vi "Actor Core.vi"(8 "error in":errorcluster, 11 "On-Grid in":refnum<class "On-Grid.lvclass">) -> (0 "error out":errorcluster, 3 "Actor out":refnum<class "Actor.lvclass">)   [LabVIEW 2018, in "On-Grid Actor.lvlib" / "On-Grid.lvclass"]
doc: "(<B>Filename</B>: Actor Framework.lvlib:Actor.lvclass:Actor Core.vi)\n\nReceives messages to the actor, reacts to them, and initiates any error handling that may shut the actor down.\n\nDescendant classes may override this VI to append parallel tasks for the actor to complete while it handles messages. Overrides use the Call Parent Method node."
uses:
  On-Grid.lvclass
  C:/Users/Administrator/Desktop/LabVIEW EMS/Optimization/Generic Optimization Actor/Generic Optimization/Generic Optimization.lvclass
  C:/Program Files (x86)/National Instruments/LabVIEW 2018/vi.lib/ActorFramework/Actor/Actor.lvclass
  C:/Users/Administrator/Desktop/LabVIEW EMS/EMS Generic Actor/EMS Generic/EMS Generic.lvclass
  <vilib>/ActorFramework/Actor/Actor.lvclass
  Generic Optimization Actor/Generic Optimization Messages/Find and Rejoin Devices Msg/Find and Rejoin Devices Msg.lvclass
  C:/Program Files (x86)/National Instruments/LabVIEW 2018/vi.lib/ActorFramework/Message/Message.lvclass
  <vilib>/ActorFramework/Actor/Actor.lvclass/Actor.ctl
  <vilib>/ActorFramework/Message Enqueuer/Message Enqueuer.lvclass/Message Enqueuer.ctl
  EMS Generic Actor/EMS Generic/EMS Generic.lvclass/EMS Generic.ctl
  Generic Optimization Actor/Generic Optimization/Optimization Controls/PCC Data.ctl
  <vilib>/ActorFramework/Message Enqueuer/Init from Existing Queue.vi
  Global Variables/Global Variables.vi
  <vilib>/ActorFramework/Message Enqueuer/Message Enqueuer.lvclass
  Generic Optimization Actor/Generic Optimization/Generic Optimization.lvclass
  EMS Generic Actor/EMS Generic/EMS Generic.lvclass
panel:
  out "Solution Result":string="Waiting"
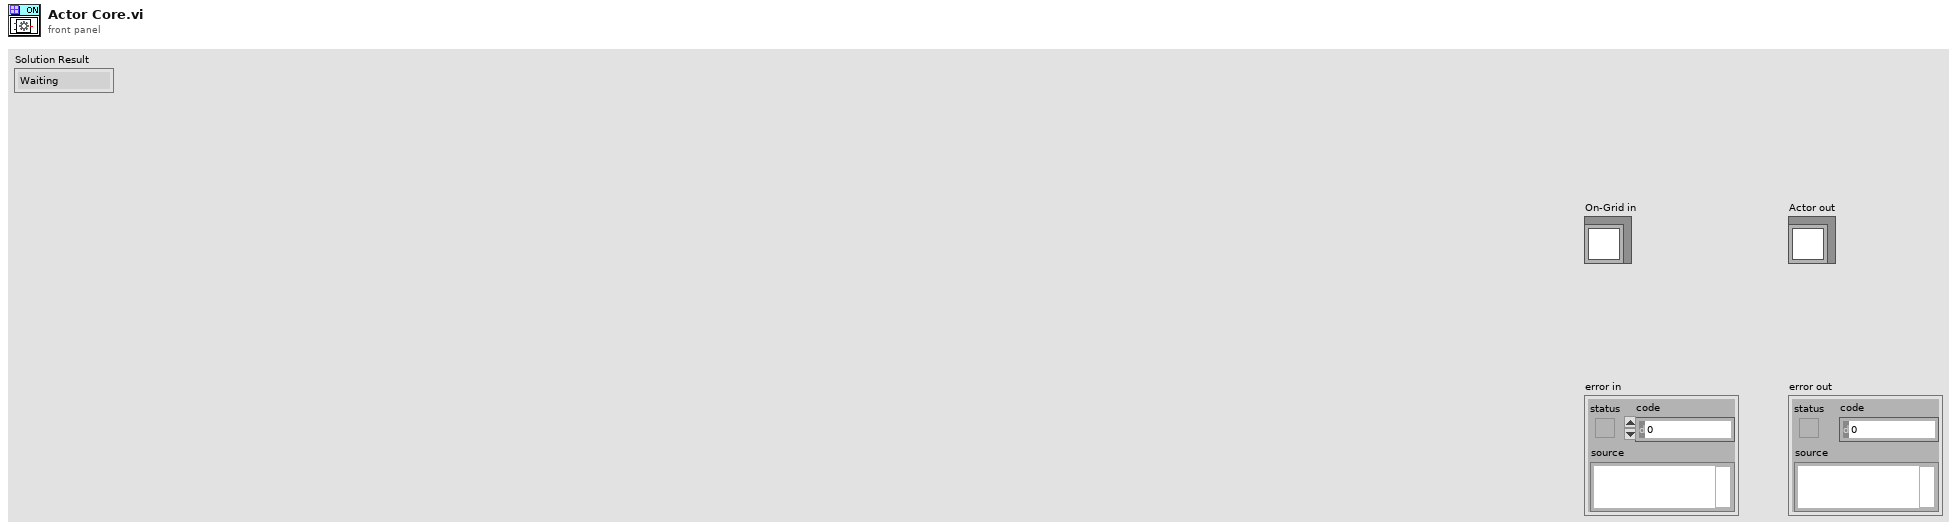
[diagram p1: front panel]
types:
  T1 = enum32{"Invalid", "Standard", "Closed", "Hidden", "Minimized", "Maximized"}
  T2 = typedef "CSEISMIC DDS.lvlib/CSEISMIC DDS.lvclass/DeviceID.ctl" = string
  T3 = typedef "Generic Optimization Actor.lvlib/Generic Optimization.lvclass/Bus by ID.ctl" = cluster{"DeviceID":T2, "Bus ID":dbl}
  T4 = typedef "Generic Optimization Actor.lvlib/Generic Optimization.lvclass/Electrical Network Optimization Data.ctl" = cluster{"From_Bus":dbl, "To_Bus":dbl, "Network Resistance":dbl, "Network Reactance":dbl, "Power Flow Limits":dbl[], "Linear Piecewise Power Flow":dbl[], "Reactive Flow Limit":dbl[], "Linear Piecewise Reactive Flow":dbl[]}
  T5 = typedef "Generic Optimization Actor.lvlib/Generic Optimization.lvclass/PCC Data.ctl" = cluster{"PCC_max":dbl[], "PCC_min":dbl[], "QCC_max":dbl[], "QCC_min":dbl[]}
  T6 = typedef "EMS Generic Actor.lvlib/EMS Generic.lvclass/Global Configuration.ctl" = cluster{"Microgrid ID":u8, "VF Device ID":T2, "Ongrid VF Priority":T2[], "Offgrid VF Priority":T2[], "AutoSwap Offgrid VF":u32, "AutoSwap Offgrid VF Delay (sec)":dbl, "AutoSwap Resynch VF":u32, "PCC Device ID":T2, "Device ID Array":T2[], "Nominal Voltage":dbl, "Nominal Frequency":dbl, "Resynch Timeout (sec)":dbl, "Island VF Activate Timeout (sec)":dbl, "Island PCC Target Power (kW)":dbl, "Island PCC Target Power Timeout (sec)":dbl, "Island Grid Settle Time (sec)":dbl, "Island PCC Failure Timeout (sec)":dbl, "Activation Devices Present Timeout (sec)":dbl, "Activation Devices Activated Timeout (sec)":dbl, "Blackstart VF GenMode Wait (sec)":dbl, "Blackstart VF DERCtrl Wait (sec)":dbl, "Blackstart Success Wait (sec)":dbl, "OnGrid Optimization Delay (sec)":dbl, "OffGrid Optimization Delay (sec)":dbl, "Resynch Frequency (Hz)":dbl, "Optimization Path":string}
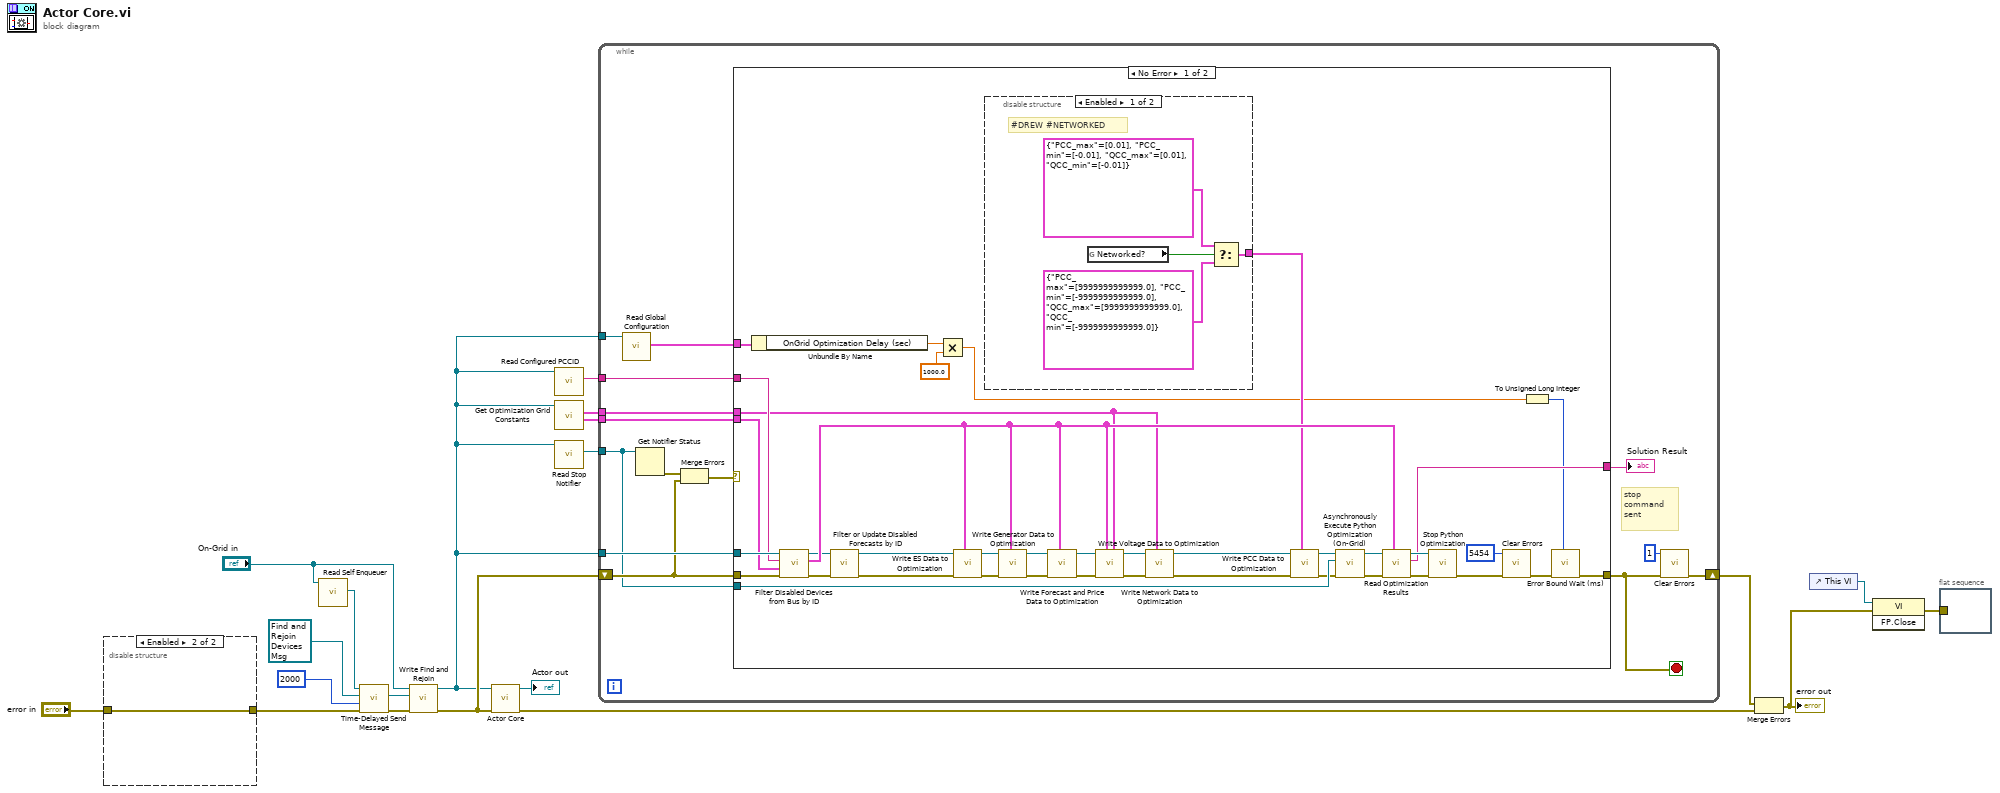
[diagram p0: block diagram]
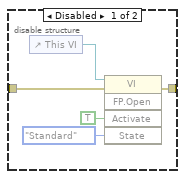
[diagram p2: hidden frame]
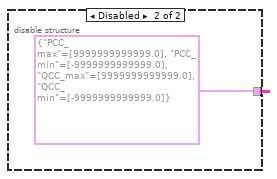
[diagram p3: hidden frame]
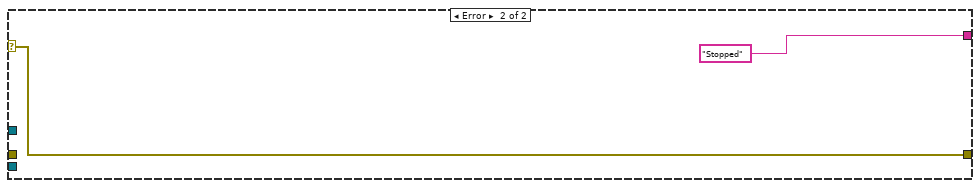
[diagram p4: hidden frame]
diagram:
  n1 = disable-structure shown="Enabled" {
    disable-tunnel: "error in" -> [w22 w26]
    disable-tunnel: [w21 w26] -> w4
    frame Disabled {
      n2 = control-ref of="This VI"() -> (w25:refnum<vi>)
      n3 = invoke class="VI" method="FP.Open"(reference=w25, error in=w22, "Activate"=TRUE ("Activate?"), "State"=T1."Standard") -> (error out=w21:errorcluster)  [unwired: 1 in, 4 out]
    }
    frame Enabled {
    }
  }
  n4 = call <vilib>:"Read Self Enqueuer.vi"("Actor"="On-Grid in") -> ("Self Enqueuer"=w9:refnum<class "Message Enqueuer.lvclass">)  [unwired: 10 in]
  n5 = call <vilib>:"Time-Delayed Send Message.vi"("error in (no error)"=w4, "Milliseconds To Wait"=2000, "Message"=refnum<class "Find and Rejoin Devices Msg.lvclass"> refnum ("Generic Optimization Actor.lvlib:Find and Rejoin Devices Msg.lvclass"), "Message Enqueuer"=w9) -> ("error out"=w7:errorcluster, "Delivery Notifier"=w6:refnum<notifier>)  [unwired: 6 in]
  n6 = call "Write Find and Rejoin.vi"("error in"=w7, "Find and Rejoin"=w6, "Generic Optimization in"="On-Grid in") -> ("error out"=w3:errorcluster, "Generic Optimization out"=w1:refnum<class "On-Grid.lvclass">)  [unwired: 7 in]
  n7 = call-parent "Actor Core.vi"("error in"=w3, "Actor in"=w1) -> ("error out"=w20:errorcluster, "Actor out"=→"Actor out":refnum<class "Actor.lvclass">)  [unwired: 8 in]
  n8 = call "Read Configured PCCID.vi"("EMS Generic in"=w1) -> ("PCCID"=w11:T2)  [unwired: 8 in, 2 out]
  n9 = call "Get Optimization Grid Constants.vi"("Generic Optimization in"=w1) -> ("Bus by ID"=w16:T3[], "Network Data"=w15:T4[])  [unwired: 8 in, 1 out]
  n10 = call "Read Stop Notifier.vi"("EMS Generic in"=w1) -> ("stop"=w18:refnum<notifier>)  [unwired: 9 in, 1 out]
  n11 = while {
    tunnel: w16 -> [w38]
    tunnel: w15 -> [w40]
    tunnel: w1 -> [w39]
    tunnel: w18 -> [w33]
    shift-right: [w30] -> w17
    shift-left: w3 -> [w35]
    tunnel: w11 -> [w29]
    tunnel: w1 -> [w28]
    stop <- w31 stop-if-true
    # "stop command sent"
    n12 = call "Read Global Configuration.vi"("EMS Generic in"=w28) -> ("Global Configuration"=w27:T6)  [unwired: 8 in, 2 out]
    n13 = Get Notifier Status(notifier=w33) -> (error out=w36:errorcluster)  [unwired: 1 in, 4 out]
    n14 = Merge Errors(w36, w35) -> (w34:errorcluster)
    n15 = case shown="No Error" w34 {
      selector: w34 -> [_ w84]
      tunnel: w40 -> [w41 _]
      tunnel: w39 -> [w58 _]
      tunnel: w35 -> [w57 _]
      tunnel: w38 -> [w56 _]
      tunnel: [w46 w84] -> w31
      tunnel: [w67 "Stopped" ("Solution Result")] -> w37
      tunnel: w33 -> [w66 _]
      tunnel: w29 -> [w55 _]
      tunnel: w27 -> [w48 _]
      frame No Error {
        n16 = Unbundle By Name(w48) -> ("OnGrid Optimization Delay (sec)"=w45:dbl)
        n17 = call "Filter Disabled Devices from Bus by ID.vi"("error in"=w57, "BusData"=w56, "PCCID"=w55, "Generic Optimization in"=w58) -> ("dup error out"=w52:errorcluster, "Filtered Bus by ID"=w54:T3[], "Generic Optimization out"=w53:refnum<class "On-Grid.lvclass">)  [unwired: 5 in]
        n18 = call "Filter or Update Disabled Forecasts by ID.vi"("error in"=w52, "Generic Optimization in"=w53) -> ("dup error out"=w51:errorcluster, "Generic Optimization out"=w50:refnum<class "On-Grid.lvclass">)  [unwired: 8 in]
        n19 = Multiply(x=w45, y=1000.0) -> (x*y=w43:dbl)
        n20 = call "Write ES Data to Optimization.vi"("Bus by ID"=w54, "error in"=w51, "Generic Optimization in"=w50) -> ("error out"=w75:errorcluster, "Generic Optimization out"=w74:refnum<class "On-Grid.lvclass">)  [unwired: 7 in]
        n21 = disable-structure shown="Enabled" {
          disable-tunnel: [w79 T5 {"PCC_max"=[9999999999999.0], "PCC_min"=[-9999999999999.0], "QCC_max"=[9999999999999.0], "QCC_min"=[-9999999999999.0]} ("PCC Data")] -> w49
          frame Enabled {
            # "#DREW #NETWORKED"
            n22 = global read "Global Variables.vi" "Networked?"() -> (w82:bool)
            n23 = Select(t=T5 {"PCC_max"=[0.01], "PCC_min"=[-0.01], "QCC_max"=[0.01], "QCC_min"=[-0.01]} ("PCC Data"), s=w82, f=T5 {"PCC_max"=[9999999999999.0], "PCC_min"=[-9999999999999.0], "QCC_max"=[9999999999999.0], "QCC_min"=[-9999999999999.0]} ("PCC Data")) -> (s? t:f=w79:T5)
          }
          frame Disabled {
          }
        }
        n24 = call "Write Generator Data to Optimization.vi"("Bus by ID"=w54, "error in"=w75, "Generic Optimization in"=w74) -> ("error out"=w78:errorcluster, "Generic Optimization out"=w73:refnum<class "On-Grid.lvclass">)  [unwired: 7 in]
        n25 = call "Write Forecast and Price Data to Optimization.vi"("Bus by ID"=w54, "error in"=w78, "Generic Optimization in"=w73) -> ("error out"=w77:errorcluster, "Generic Optimization out"=w72:refnum<class "On-Grid.lvclass">)  [unwired: 7 in]
        n26 = call "Write Voltage Data to Optimization.vi"("Network Data Array"=w41, "Bus by ID"=w54, "error in"=w77, "Generic Optimization in"=w72) -> ("error out"=w76:errorcluster, "Generic Optimization out"=w71:refnum<class "On-Grid.lvclass">)  [unwired: 6 in]
        n27 = call "Write Network Data to Optimization.vi"("Network Data Array"=w41, "error in"=w76, "Generic Optimization in"=w71) -> ("error out"=w65:errorcluster, "Generic Optimization out"=w64:refnum<class "On-Grid.lvclass">)  [unwired: 7 in]
        n28 = call "Write PCC Data to Optimization.vi"("PCC Data"=w49, "error in"=w65, "Generic Optimization in"=w64) -> ("error out"=w62:errorcluster, "Generic Optimization out"=w60:refnum<class "On-Grid.lvclass">)  [unwired: 7 in]
        n29 = call "Asynchronously Execute Python Optimization (On-Grid).vi"("error in"=w62, "Stop Notifier"=w66, "On-Grid in"=w60) -> ("error out"=w59:errorcluster, "On-Grid out"=w61:refnum<class "On-Grid.lvclass">)  [unwired: 7 in]
        n30 = call "Read Optimization Results.vi"("Bus by ID Array"=w54, "error in"=w59, "Generic Optimization in"=w61) -> ("error out"=w69:errorcluster, "Solution Result"=w67:string, "Generic Optimization out"=w70:refnum<class "On-Grid.lvclass">)  [unwired: 6 in]
        n31 = call "Stop Python Optimization.vi"("error in"=w69, "Generic Optimization in"=w70) -> ("error out"=w63:errorcluster)  [unwired: 8 in, 1 out]
        n32 = call <vilib>:"Clear Errors.vi"("error in (no error)"=w63, "specific error code to clear (0: all)"=5454) -> ("error out"=w47:errorcluster)  [unwired: 4 in, 1 out]
        n33 = To Unsigned Long Integer(number=w43) -> (unsigned 32bit integer=w42:u32)
        n34 = call "Error Bound Wait (ms).vi"("milliseconds to wait (100)"=w42, "error in"=w47) -> ("error out"=w46:errorcluster)  [unwired: 9 in]
      }
      frame Error {
      }
    }
    "Solution Result" <- w37
    n35 = call <vilib>:"Clear Errors.vi"("error in (no error)"=w31, "specific error code to clear (0: all)"=1) -> ("error out"=w30:errorcluster)  [unwired: 4 in, 1 out]
  }
  n36 = Merge Errors(w17, w20) -> (w13:errorcluster)
  "error out" <- w13
  n37 = control-ref of="This VI"() -> (w14:refnum<vi>)
  n38 = invoke class="VI" method="FP.Close"(reference=w14, error in=w13) -> (error out=w12:errorcluster)  [unwired: 1 in, 2 out]
  n39 = flat-sequence {
    tunnel: w12 -> [_]
    frame #0 {
    }
  }
